vi "Set all delays.vi"(8 "error in (no error)":errorcluster, 11 "Sync Box in":refnum<class "Sync Box.lvclass">) -> (0 "error out":errorcluster, 3 "Sync Box out":refnum<class "Sync Box.lvclass">)   [LabVIEW 2018, in "Sync Box.lvclass"]
uses:
  Sync Box.lvclass
panel:
  in  "Set all delays":string
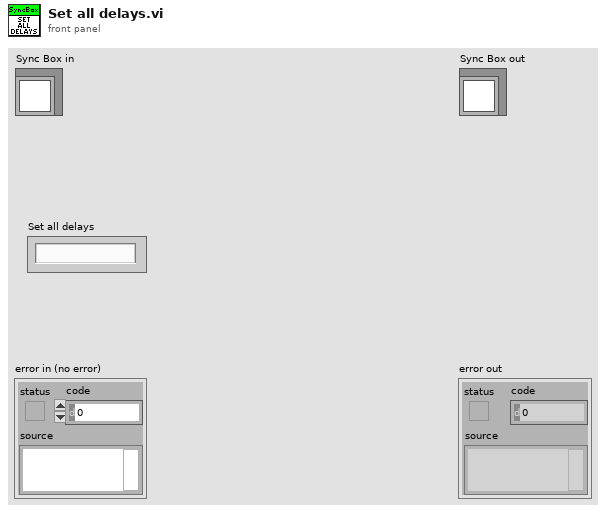
[diagram p1: front panel]
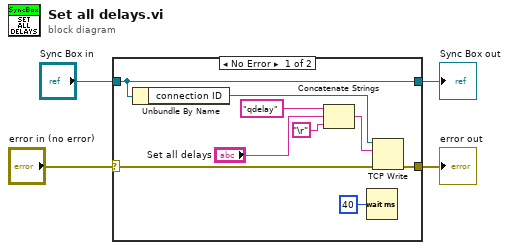
[diagram p0: block diagram]
diagram:
  n1 = case shown="No Error" "error in (no error)" {
    selector: "error in (no error)" -> [w11 w15]
    tunnel: [w10 w15] -> w1
    tunnel: "Sync Box in" -> [w7 w14]
    tunnel: [w7 w14] -> w2
    frame No Error {
      n2 = Unbundle By Name(w7) -> ("connection ID"=w8:refnum<k5>)
      n3 = Concatenate Strings("qdelay", "Set all delays", "\r") -> (w13:string)
      n4 = Wait (ms)(milliseconds to wait=u32 40) -> ()  [unwired: 1 out]
      n5 = TCP Write(connection ID=w8, data in=w13, error in (no error)=w11) -> (error out=w10:errorcluster)  [unwired: 1 in, 2 out]
    }
    frame Error {
    }
  }
  "error out" <- w1
  "Sync Box out" <- w2
